vi "Write current unit ID.vi"(8 "error in (no error)":errorcluster, 10 "request unit ID":u8, 11 "serial data unit in":refnum<class "Serial Data Unit.lvclass">) -> (0 "error out":errorcluster, 3 "serial data unit out":refnum<class "Serial Data Unit.lvclass">)   [LabVIEW 2020, in "SubVIs.lvlib" / "Serial Data Unit.lvclass"]
uses:
  <vilib>/Modbus/subvis/Transmission Data Unit (ADU)/Serial Data Unit/Serial Data Unit.lvclass
  <vilib>/Modbus/subvis/Transmission Data Unit (ADU)/Serial Data Unit/Serial Data Unit.lvclass/Serial Data Unit.ctl
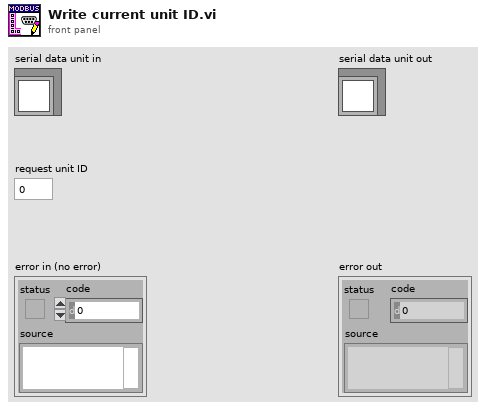
[diagram p1: front panel]
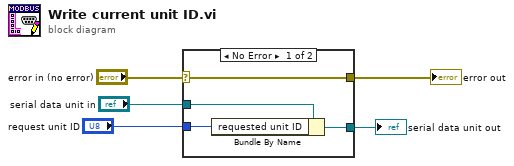
[diagram p0: block diagram]
diagram:
  n1 = case shown="No Error" "error in (no error)" {
    selector: "error in (no error)" -> [w9 w10]
    tunnel: [w9 w10] -> w4
    tunnel: [w7 w11] -> w2
    tunnel: "serial data unit in" -> [w8 w11]
    tunnel: "request unit ID" -> [w6 _]
    frame No Error {
      n2 = Bundle By Name(cluster=w8, "requested unit ID"=w6) -> (w7:refnum<class "Serial Data Unit.lvclass">)
    }
    frame Error {
    }
  }
  "error out" <- w4
  "serial data unit out" <- w2
